vi "Draw Wrkspc Velocity.vi"(6 "velocities":dbl[][](array[numeric]), 7 "name":string, 8 "error in (no error)":errorcluster, 9 "workspace in":dbl[][](array[numeric]), 10 "parent sence":refnum<vi>, 11 "Delta Analyzor in":refnum<class "Delta Analyzor.lvclass">) -> (0 "error out":errorcluster, 1 "Wrkspc vel Obj":refnum<vi>, 2 "parent sence out":refnum<vi>, 3 "Delta Analyzor out":refnum<class "Delta Analyzor.lvclass">)   [LabVIEW 2013, in "Delta Analyzor.lvclass"]
uses:
  Delta Analyzor.lvclass
  <vilib>/Utility/miscctls.llb/LV3DPointTypeDef.ctl
  <vilib>/Utility/miscctls.llb/LVRGBAColorTypeDef.ctl
  <vilib>/Analysis/_algsub.llb/Real Vector Norm.vi
  <vilib>/picture/3D Picture Control/Object/Create Object (name).vi
  <vilib>/picture/3D Picture Control/NI_3D Picture Control.lvlib
  <vilib>/Analysis/NI_AALPro.lvlib
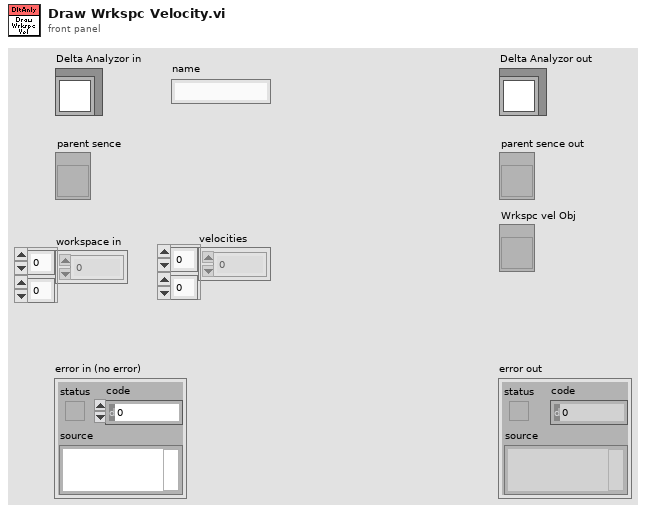
[diagram p1: front panel]
types:
  T1 = typedef "LV3DPointTypeDef.ctl" = cluster{"X":sgl, "Y":sgl, "Z":sgl}
  T2 = enum16{"Overall", "Per Primitive", "Per Vertex", "Binding Off"}
  T3 = enum16{"Points", "Lines", "Line Strip", "Line Loop", "Triangles", "Triangle Strip", "Triangle Fan", "Quads", "Quad Strip", "Polygon"}
  T4 = typedef "LVRGBAColorTypeDef.ctl" = cluster{"Red":sgl, "Green":sgl, "Blue":sgl, "Alpha":sgl}
  T5 = cluster{"velocities[0]":dbl, "velocities[1]":dbl, "velocities[2]":dbl}
  T6 = cluster{"workspace in[0]":dbl, "workspace in[1]":dbl, "workspace in[2]":dbl}
  T7 = cluster{"workspace in[0]":dbl, "workspace in[1]":dbl, "workspace in[2]":dbl}[]
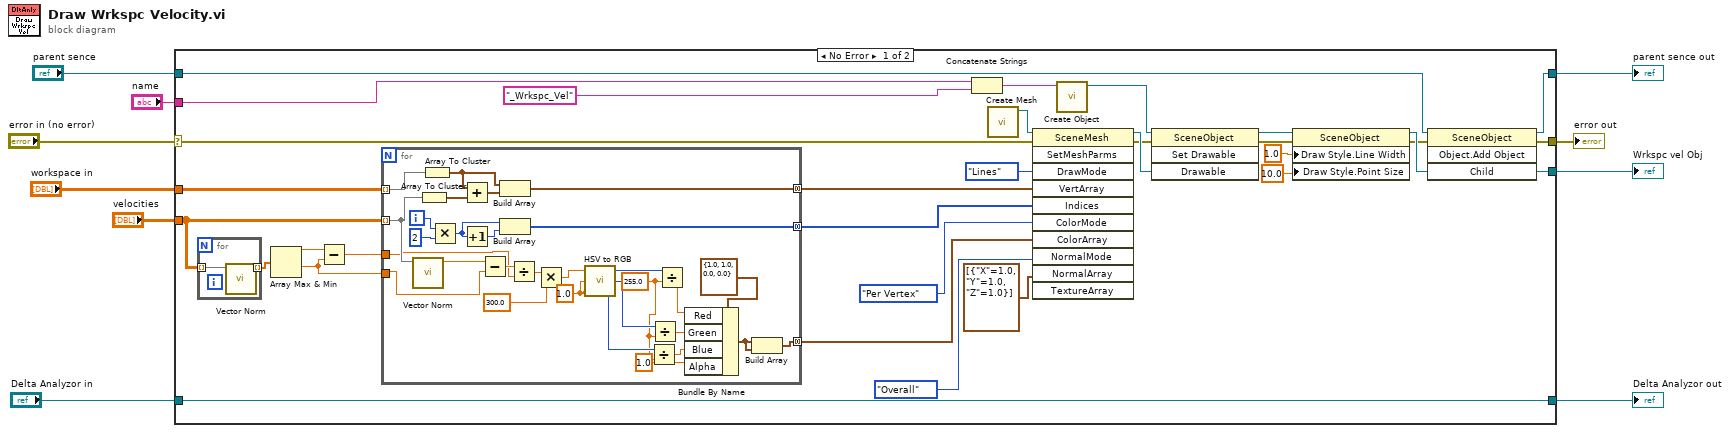
[diagram p0: block diagram]
diagram:
  n1 = case shown="No Error" "error in (no error)" {
    selector: "error in (no error)" -> [w23 w77]
    tunnel: [w19 w77] -> w9
    tunnel: [w42 w76] -> w7
    tunnel: "Delta Analyzor in" -> [w42 w76]
    tunnel: "workspace in" -> [w39 _]
    tunnel: "velocities" -> [w15 _]
    tunnel: "name" -> [w32 _]
    tunnel: "parent sence" -> [w30 w75]
    tunnel: [w29 w75] -> w2
    tunnel: [w28 _] -> w1
    frame No Error {
      n2 = for {
        tunnel: w15 -> [w44] mode=indexing
        tunnel: [w43] -> w14 mode=indexing
        n3 = call-poly <vilib>:"Vector Norm.vi"("Input Vector"=w44) -> ("norm"=w43:dbl)  [unwired: 9 in, 1 out]
      }
      n4 = Array Max & Min(array=w14) -> (max value=w16:dbl, min value=w12:dbl)  [unwired: 2 out]
      n5 = Subtract(x=w16, y=w12) -> (x-y=w13:dbl)
      n6 = for {
        tunnel: w39 -> [w74] mode=indexing
        tunnel: w15 -> [w64] mode=indexing
        tunnel: [w70] -> w38 mode=concatenating
        tunnel: [w65] -> w37 mode=concatenating
        tunnel: w13 -> [w48]
        tunnel: w12 -> [w49]
        tunnel: [w45] -> w11 mode=concatenating
        i -> [w69]
        w53 = 255.0
        w62 = 1.0 ("S")
        n7 = call-poly <vilib>:"Vector Norm.vi"("Input Vector"=w64) -> ("norm"=w50:dbl)  [unwired: 9 in, 1 out]
        n8 = Array To Cluster(array=w64) -> (cluster=w73:T5)
        n9 = Array To Cluster(array=w74) -> (cluster=w71:T6)
        n10 = Multiply(x=w69, y=2) -> (x*y=w66:i32)
        n11 = Add(x=w71, y=w73) -> (x+y=w72:cluster{dbl, dbl, dbl})
        n12 = Increment(x=w66) -> (x+1=w67:i32)
        n13 = Subtract(x=w50, y=w49) -> (x-y=w63:dbl)
        n14 = Build Array(w71, w72) -> (w70:T7)
        n15 = Build Array(w66, w67) -> (w65:i32[])
        n16 = Divide(x=w63, y=w48) -> (x/y=w61:dbl)
        n17 = Multiply(x=w61, y=300.0) -> (x*y=w59:dbl)
        n18 = call "HSV to RGB.vi"("V"=w62, "S"=w62, "H"=w59) -> ("B"=w54:u8, "G"=w56:u8, "R"=w58:u8)
        n19 = Divide(x=w54, y=w53) -> (x/y=w52:dbl)
        n20 = Divide(x=w56, y=w53) -> (x/y=w55:dbl)
        n21 = Divide(x=w58, y=w53) -> (x/y=w57:dbl)
        n22 = Bundle By Name(cluster=T4 {"Red"=1.0, "Green"=1.0, "Blue"=0.0, "Alpha"=0.0} ("Color"), "Red"=w57, "Green"=w55, "Blue"=w52, "Alpha"=sgl 1.0) -> (w46:T4)
        n23 = Build Array(w46, w46) -> (w45:T4[])
      }
      n24 = Concatenate Strings(w32, "_Wrkspc_Vel" ("string")) -> (w33:string)
      n25 = call <vilib>:"Create Mesh.vi"() -> ("New Mesh Refnum"=w41:refnum<vi>)  [unwired: 10 in, 1 out]
      n26 = invoke class="SceneMesh" method="SetMeshParms"(reference=w41, error in=w23, "DrawMode"=T3."Lines" ("Draw Mode"), "VertArray"=w38, "Indices"=w37, "ColorMode"=T2."Per Vertex" ("Color Binding Mode"), "ColorArray"=w11, "NormalMode"=T2."Overall" ("Normal Binding Mode"), "NormalArray"=T1[] [{"X"=1.0, "Y"=1.0, "Z"=1.0}] ("Normal Array")) -> (reference out=w31:refnum<vi>, error out=w22:errorcluster)  [unwired: 2 in, 9 out]
      n27 = call-poly <vilib>:"Create Object.vi"("Name"=w33) -> ("Scene:New Object"=w27:refnum<vi>)  [unwired: 9 in, 1 out]
      n28 = invoke class="SceneObject" method="Set Drawable"(reference=w27, error in=w22, "Drawable"=w31) -> (reference out=w26:refnum<vi>, error out=w21:errorcluster)  [unwired: 1 in, 2 out]
      n29 = property class="SceneObject"(reference=w26, error in=w21, "Draw Style.Line Width"=sgl 1.0 ("Draw Style:Line Width"), "Draw Style.Point Size"=sgl 10.0 ("Draw Style:Point Size")) -> (reference out=w24:refnum<vi>, error out=w20:errorcluster)
      n30 = invoke class="SceneObject" method="Object.Add Object"(reference=w30, error in=w20, "Child"=w24) -> (reference out=w29:refnum<vi>, error out=w19:errorcluster, "Child"=w28:refnum<vi>)  [unwired: 1 in, 1 out]
    }
    frame Error {
    }
  }
  "error out" <- w9
  "Delta Analyzor out" <- w7
  "Wrkspc vel Obj" <- w1
  "parent sence out" <- w2
